vi "sub_usb_hw-list.vi"(10 "Password":string, 11 "User Name":string) -> (3 "Resources":string[][](table))   [LabVIEW 2019]
uses:
  <vilib>/Utility/error.llb/DialogType.ctl
  <vilib>/nisyscfg/Filter Mode.ctl
  <vilib>/nisyscfg/Close (Hardware).vi
  <vilib>/nisyscfg/Close (Filter).vi
  <vilib>/nisyscfg/Close (System).vi
  <resource>/objmgr/nicontrollersysapi.rc
  <vilib>/nisyscfg/nisyscfg.lvlib
panel:
  in  "Target (localhost)":refnum<k21>="localhost"
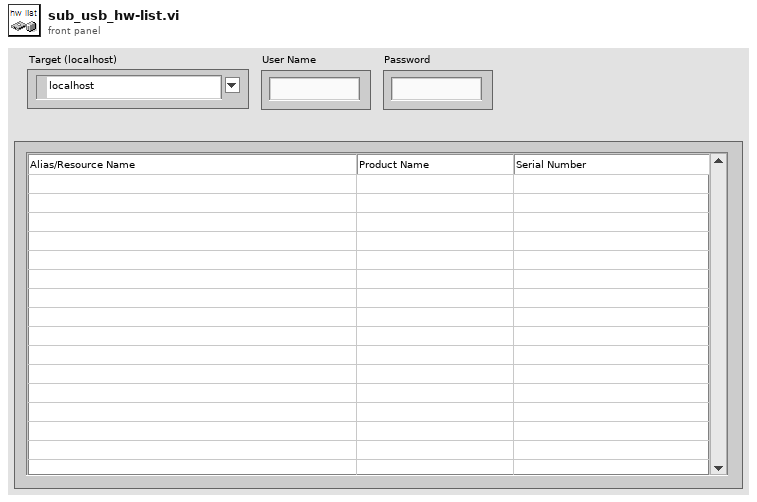
[diagram p1: front panel]
types:
  T1 = typedef "nisyscfg.lvlib/Filter Mode.ctl" = i32
  T2 = typedef "DialogType.ctl" = u16
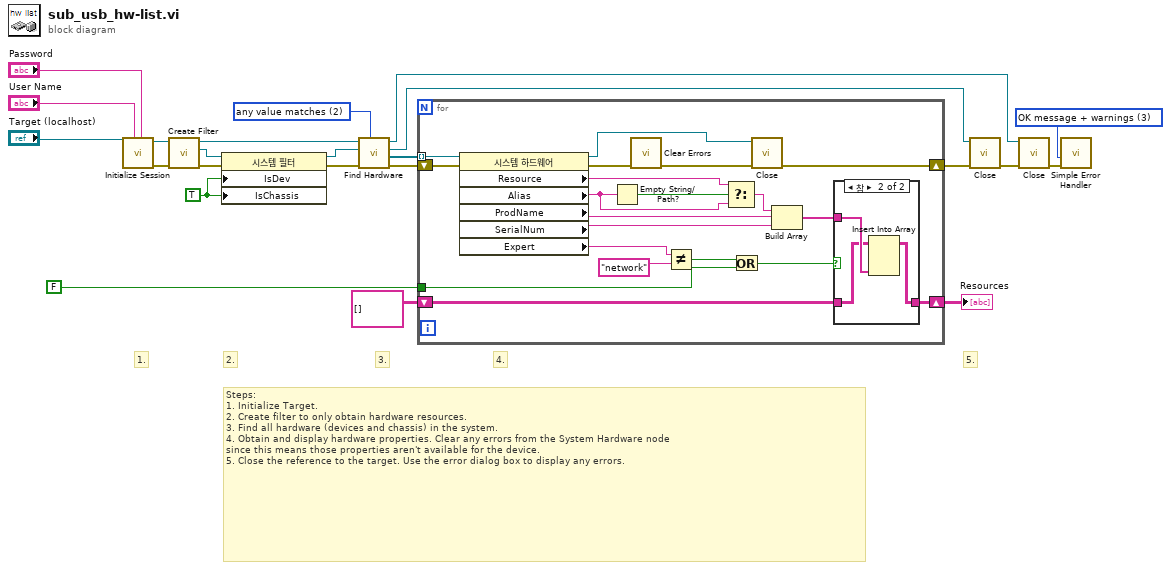
[diagram p0: block diagram]
diagram:
  w9 = T1 2 items=["all values match"=1, "any value matches"=2, "values do not match"=3, "all properties exist"=4] ("filter mode (all values match)")
  w1 = TRUE ("Is Chassis")
  w17 = T2 3 items=["no dialog", "OK message", "continue or stop message", "OK message + warnings", "continue/stop + warnings"] ("type of dialog (OK msg:1)")
  # "2."
  # "5."
  # "4."
  # "3."
  # "1."
  # "Steps:\n1. Initialize Target.\n2. Create filter to only obtain hardware resources.\n3. Find all hardware (devices and chassis) in the system.\n4. Obtain and display hardware properties. Clear any errors from the System Hardware node\nsince this means those properties aren't available for the device. \n5. Close the reference to the target. Use the error dialog box to display any errors."
  n1 = call <vilib>:"Initialize Session.vi"("Password"="Password", "User Name"="User Name", "Target (localhost)"="Target (localhost)") -> ("error out"=w11:errorcluster, "Session out"=w14:refnum<k21>)  [unwired: 7 in]
  n2 = call <vilib>:"Create Filter.vi"("error in (no error)"=w11, "Session in"=w14) -> ("error out"=w16:errorcluster, "Filter out"=w15:refnum<k20>, "Session out"=w13:refnum<k21>)  [unwired: 7 in]
  n3 = property class="시스템 필터"(reference=w15, error in=w16, "IsDev"=w1, "IsChassis"=w1) -> (reference out=w10:refnum<k20>, error out=w12:errorcluster)
  n4 = call <vilib>:"Find Hardware.vi"("Filter Mode (all values match)"=w9, "error in (no error)"=w12, "Filter in"=w10, "Session in"=w13) -> ("error out"=w5:errorcluster, "Resources out"=w23:refnum<k20>[], "Filter out"=w7:refnum<k20>, "Session out"=w18:refnum<k21>)  [unwired: 4 out]
  n5 = for {
    tunnel: w23 -> [w41] mode=indexing
    shift-right: [w43] -> w6
    shift-left: w5 -> [w33]
    shift-right: [w32] -> w20
    shift-left: string[][] [] ("Results") -> [w30]
    tunnel: FALSE ("Show All Network Devices") -> [w25]
    n6 = property class="시스템 하드웨어"(reference=w41, error in=w33) -> (reference out=w34:refnum<k20>, error out=w35:errorcluster, "Resource"=w39:string, "Alias"=w40:string, "ProdName"=w37:string, "SerialNum"=w36:string, "Expert"=w29:string)
    n7 = Empty String/Path?(string/path=w40) -> (empty?=w42:bool)
    n8 = call <vilib>:"Clear Errors.vi"("error in (no error)"=w35) -> ("error out"=w24:errorcluster)  [unwired: 5 in, 1 out]
    n9 = Not Equal?(x=w29, y="network") -> (x != y?=w26:bool)
    n10 = Select(t=w39, s=w42, f=w40) -> (s? t:f=w38:string)
    n11 = Or(x=w26, y=w25) -> (x .or. y?=w27:bool)
    n12 = call-poly <vilib>:"Close.vi"("error in (no error)"=w24, "Resource in"=w34) -> ("error out"=w43:errorcluster)  [unwired: 9 in]
    n13 = Build Array(w38, w37, w36) -> (w31:string[])
    n14 = case shown="참" w27 {
      tunnel: [w44 w47] -> w32
      tunnel: w31 -> [_ w46]
      tunnel: w30 -> [w44 w45]
      frame False {
      }
      frame True {
        n15 = Insert Into Array(array=w45, new element=w46) -> (w47:string[][])  [unwired: 2 in]
      }
    }
  }
  "Resources" <- w20
  n16 = call-poly <vilib>:"Close.vi"("error in (no error)"=w6, "Filter in"=w7) -> ("error out"=w8:errorcluster)  [unwired: 9 in]
  n17 = call-poly <vilib>:"Close.vi"("error in (no error)"=w8, "Session in"=w18) -> ("error out"=w22:errorcluster)  [unwired: 9 in]
  n18 = call <vilib>:"Simple Error Handler.vi"("type of dialog (OK msg:1)"=w17, "error in (no error)"=w22) -> ()  [unwired: 3 in, 5 out]
